vi "LHS and RHS Y Scale.vi"(10 "Numeric":i32, 11 "Selected Variables":string[](array[string])) -> (3 "Array":bool[](array[boolean]))   [LabVIEW 2013]
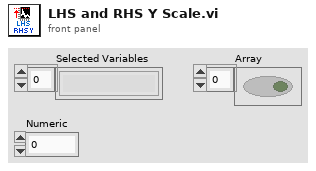
[diagram p1: front panel]
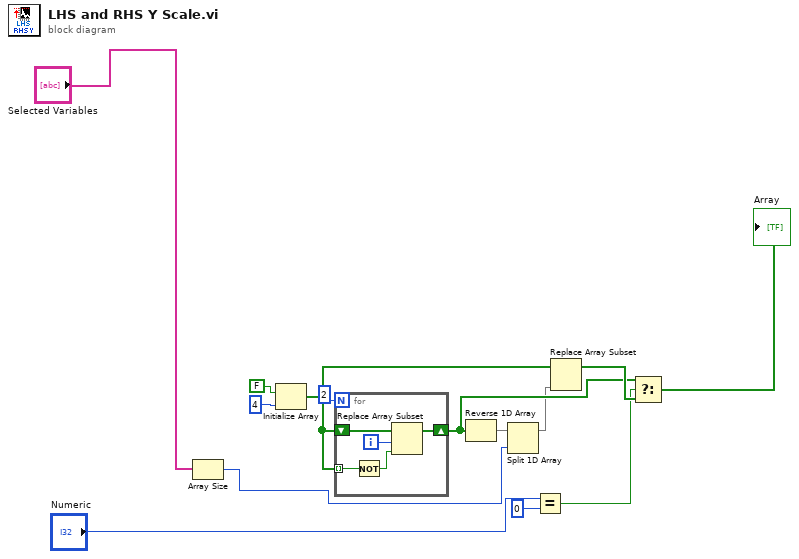
[diagram p0: block diagram]
diagram:
  n1 = Array Size(array="Selected Variables") -> (size(s)=w12:i32)
  n2 = Initialize Array(FALSE, 4 ("dimension size")) -> (w10:bool[])
  n3 = for {
    N: 2 -> [_]
    tunnel: w10 -> [w19] mode=indexing
    shift-right: [w15] -> w13
    shift-left: w10 -> [w18]
    i -> [w17]
    n4 = Not(x=w19) -> (.not. x?=w16:bool)
    n5 = Replace Array Subset(array=w18, new element=w16, index=w17) -> (w15:bool[])
  }
  n6 = Reverse 1D Array(array=w13) -> (reversed array=w9:bool[])
  n7 = Split 1D Array(array=w9, index=w12) -> (first subarray=w11:bool[])  [unwired: 1 out]
  n8 = Equal?(x="Numeric", y=0) -> (x = y?=w5:bool)
  n9 = Replace Array Subset(array=w10, new element=w11) -> (w14:bool[])  [unwired: 1 in]
  n10 = Select(t=w13, s=w5, f=w14) -> (s? t:f=→"Array":bool[])
